vi "Reset Aborted.vi"(8 "error in (no error)":errorcluster, 11 "Test Runner In":refnum<class "Test Runner.lvclass">) -> (0 "error out":errorcluster, 3 "Test Runner Out":refnum<class "Test Runner.lvclass">)   [LabVIEW 2020, in "Test Runner.lvclass"]
doc: "Resets the abort notifier."
uses:
  Test Runner.lvclass
  Test Runner.lvclass/Test Runner.ctl
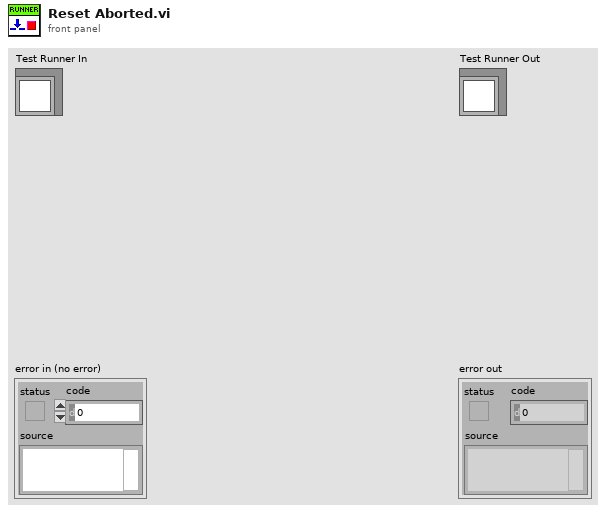
[diagram p1: front panel]
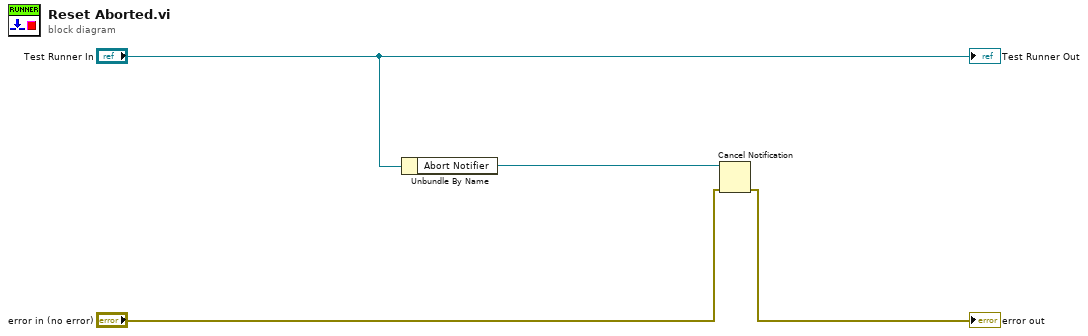
[diagram p0: block diagram]
diagram:
  n1 = Unbundle By Name("Test Runner In") -> ("Abort Notifier"=w3:refnum<notifier>)
  n2 = Cancel Notification(0:w3, 3:"error in (no error)") -> (11:→"error out":errorcluster)  [unwired: 2 out]
  "Test Runner Out" <- "Test Runner In"
